vi "logee.vi"() -> ()   [LabVIEW 2020]
panel:
  out "String":string
  out "Rouded Value":dbl
  in  "VISA resource name":refnum<visa-resource-name>
  in  "stop 2":bool
  out "Voltage signal":dbl
  out "FSR outputs":dynamicdata(graph)
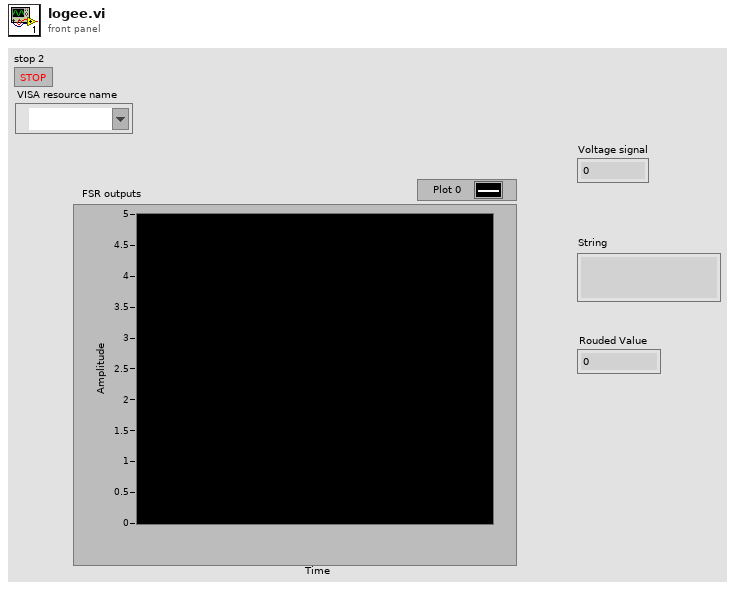
[diagram p1: front panel]
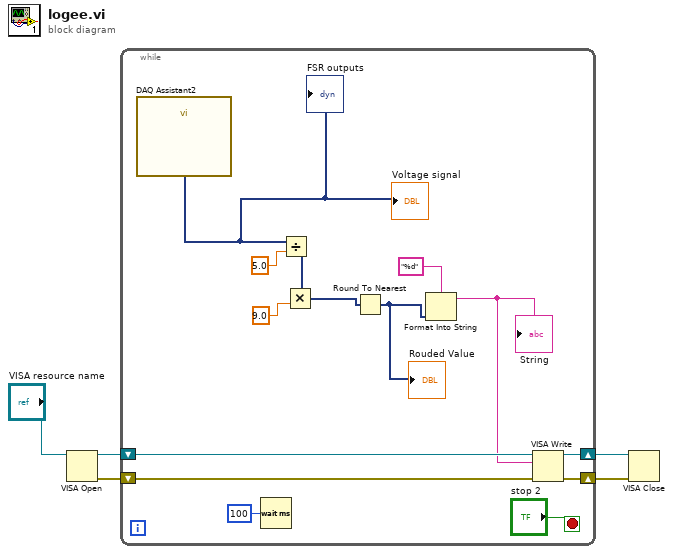
[diagram p0: block diagram]
diagram:
  n1 = VISA Open(VISA resource name="VISA resource name") -> (VISA resource name=w5:refnum<visa-resource-name>, error out=w4:errorcluster)  [unwired: 4 in]
  n2 = while {
    shift-right: [w12] -> w3
    shift-left: w5 -> [w14]
    shift-right: [w11] -> w2
    shift-left: w4 -> [w13]
    stop <- "stop 2" stop-if-true
    n3 = call "DAQ Assistant2"() -> ("data"=w15:dynamicdata)  [unwired: 17 in, 2 out]
    "FSR outputs" <- w15
    "Voltage signal" <- w15
    n4 = Wait (ms)(milliseconds to wait=u32 100) -> ()  [unwired: 1 out]
    n5 = Divide(x=w15, y=5.0) -> (x/y=w18:dynamicdata)
    n6 = Multiply(x=w18, y=9.0) -> (x*y=w16:dynamicdata)
    n7 = Round To Nearest(number=w16) -> (nearest integer value=w8:dynamicdata)
    "Rouded Value" <- w8
    n8 = Format Into String(format string="%d", w8) -> (resulting string=w6:string)  [unwired: 2 in, 1 out]
    "String" <- w6
    n9 = VISA Write(VISA resource name=w14, write buffer=w6, error in (no error)=w13) -> (VISA resource name out=w12:refnum<visa-resource-name>, error out=w11:errorcluster)  [unwired: 1 out]
  }
  n10 = VISA Close(VISA resource name=w3, error in (no error)=w2) -> ()  [unwired: 1 out]
